vi "Real-time clock accuracy measu.vi"(8 "error in":errorcluster) -> (0 "error out":errorcluster, 1 "Pass/Fail":bool, 2 "Tlcu Temp":dbl format="%#_12f", 3 "MeasuredFreq":string, 5 "Adjustment factor":string)   [LabVIEW 2009]
uses:
  Digit IO PCI 6503/Digit IO control.ctl
  Global/Global 1.vi
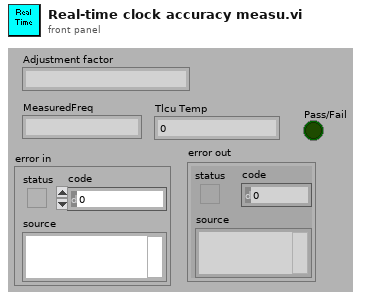
[diagram p1: front panel]
types:
  T1 = typedef "Digit IO control.ctl" = enum16{"Pull X1_4 Low", "Disconnect Pull X1_4 Low", "Down Cylinder", "Disconnect Down Cylinder", "Load X1_1_5", "Disconnect Load X1_1_5", "Measu X1_1_5", "Disconnect Measu X1_1_5", "Measu Z1_1_5", "Disconnect Measu Z1_1_5", "Power X1_1", "Disconnect Power X1_1", "RS232 Power", "Disconnect RS232 Power", "Card Cylinder", "Disconnect Card Cylinder", "Fail LED", "Disconnect Fail LED", "LCA Power", "Disconnect LCA Power", "BeyondCylinderDowndigit", "Disconnect BeyondCylinderDowendigit", "Frequency", "Disconnect Frequency", "Measu Current", "Disconnect Measu Current", "Measu current_1", "Disconnect Measu current_1", "Digit ALL", "Disconnect Digit ALL", "PASS LED", "Disconnect PASS LED", "Load Z1_1_3", "Disconnect Load Z1_1_3", "RS232 Connect", "Disconnect RS232 Connect", "Power Z1_7", "Disconnect Power Z1_7", "Pull Z_1_5  low", "Disconnect Pull Z_1_5  low", "Connect LCA_1", "Disconnect LCA_1", "short LCA", "Disconnect short LCA", "PT100", "Disconnect PT100", "NO connect", "Disconnect NO connect"}
  T2 = cluster{"People":string, "product  number":string, "Test time":string, "VHeatFuse_noload":string, "VHeatFuse_load":string, "VoverrideDiode":string, "Test firmware upload via X1":string, "TemperAddress":string, "Troom":string, "TLCU":string, "Adjustment factor":string, "MeasuredFreq":string, "I2C communication":string, "Light-emitting diode on Z2":string, "Battery warning/inhibit":string, "Reset by IC10":string, "External EEPROM":string, "RFID card detection and reading RFID":string, "Production parameters in internal EEPROM":string, "Current consumption in sleep mode":string, "Application and database upload":string, "Test result":string, "Table head[22]":string, "Table head[23]":string}
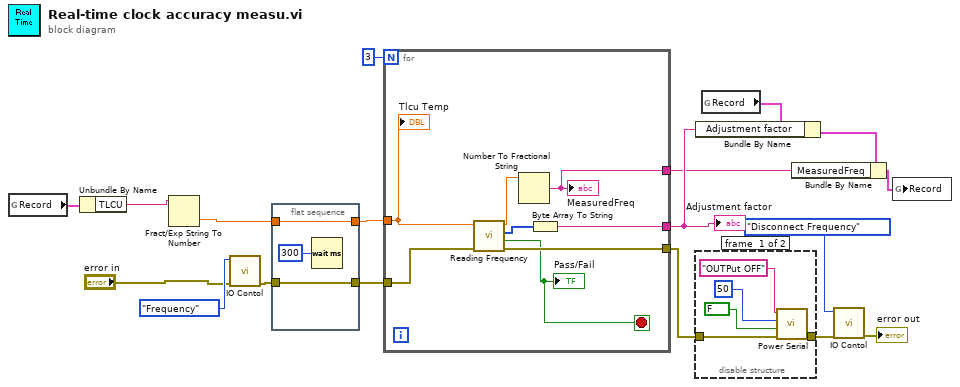
[diagram p0: block diagram]
diagram:
  n1 = global read "Global 1.vi" "Record"() -> (w4:T2)
  n2 = Unbundle By Name(w4) -> ("TLCU"=w3:string)
  n3 = Fract/Exp String To Number(string=w3) -> (number=w1:dbl)  [unwired: 4 out]
  n4 = call "IO Contol.vi"("error in"="error in", "IO Operation"=Digit_IO_control."Frequency" ("Enum")) -> ("error out"=w13:errorcluster)  [unwired: 9 out]
  n5 = flat-sequence {
    tunnel: [w20] -> w12
    tunnel: w13 -> [w20]
    tunnel: w1 -> [w19]
    tunnel: [w19] -> w11
    frame #0 {
      n6 = Wait (ms)(milliseconds to wait=u32 300) -> ()  [unwired: 1 out]
    }
  }
  n7 = for {
    N: 3 -> [_]
    tunnel: w12 -> [w29]
    tunnel: w11 -> [w28]
    tunnel: [w27] -> w15
    tunnel: [w24] -> w8
    tunnel: [w22] -> w5
    stop <- w25 stop-if-true
    n8 = call "Reading Frequency.vi"("error in"=w29, "Tlcu Temp"=w28) -> ("Error Out"=w27:errorcluster, "Pass/Fail"=w25:bool, "Adj Factor"=w26:u8[], "MeasuredFreq_1"=w23:dbl)  [unwired: 6 out]
    "Pass/Fail" <- w25
    n9 = Number To Fractional String(number=w23) -> (F-format string=w22:string)  [unwired: 3 out]
    "MeasuredFreq" <- w22
    n10 = Byte Array To String(unsigned byte array=w26) -> (string=w24:string)
    "Tlcu Temp" <- w28
  }
  "Adjustment factor" <- w8
  n11 = disable-structure shown="Enabled" {
    disable-tunnel: [w34 w35] -> w17
    disable-tunnel: w15 -> [w33 w35]
    frame #0 {
      n12 = call "Power Serial.vi"("error in (no error)"=w33, "Rd?"=FALSE, "Delay"=50, "IN"="OUTPut OFF" ("In")) -> ("error out"=w34:errorcluster)  [unwired: 6 in, 1 out]
    }
    frame #1 {
    }
  }
  n13 = global read "Global 1.vi" "Record"() -> (w9:T2)
  n14 = Bundle By Name(cluster=w9, "Adjustment factor"=w8) -> (w7:T2)
  n15 = Bundle By Name(cluster=w7, "MeasuredFreq"=w5) -> (w6:T2)
  n16 = call "IO Contol.vi"("error in"=w17, "IO Operation"=Digit_IO_control."Disconnect Frequency" ("Enum")) -> ("error out"=→"error out":errorcluster)  [unwired: 9 out]
  n17 = global write "Global 1.vi" "Record"(w6) -> ()
